vi "Opt_ROI.vi"(8 "error in (no error)":errorcluster, 10 "Number of Pre-Process Frames":i32, 11 "LTRBC":dbl[][](array[numeric])) -> (0 "error out":errorcluster, 2 "Y Centroid":dbl, 3 "ROI Out":T1 {"Contours"."Type" items=["No Selection", "Point", "Line", "Rectangle", "Oval", "Polygon", "Freehand Region", "Annulus", "Unused2", "Unused3", "Broken Line", "Freehand Line", "Rotated Rectangle"]})   [LabVIEW 2014]
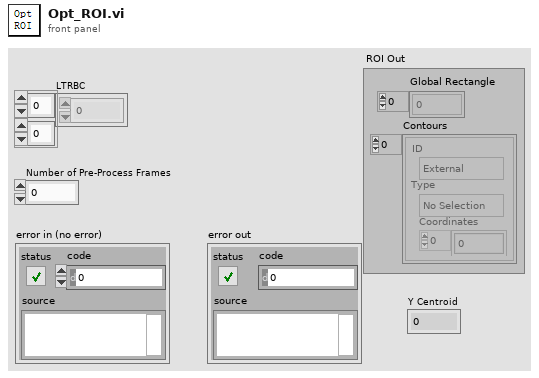
[diagram p1: front panel]
types:
  T1 = typedef "ROI Descriptor" = cluster{"Global Rectangle":i32[], "Contours":cluster{"ID":enum32{"External", "Internal"}, "Type":u32, "Coordinates":i32[]}[]}
  T2 = typedef "IMAQ Rectangle" = cluster{"Left":i32, "Top":i32, "Right":i32, "Bottom":i32, "Rotation":dbl}
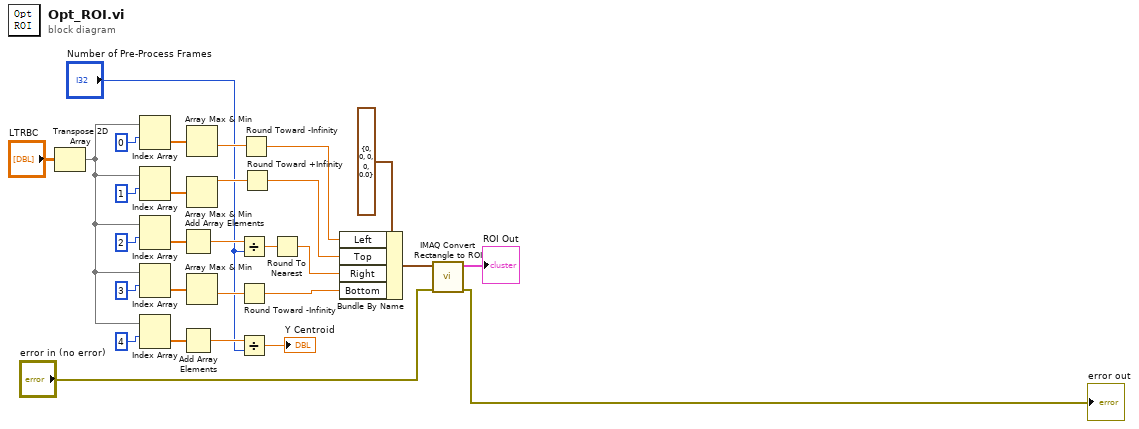
[diagram p0: block diagram]
diagram:
  n1 = Transpose 2D Array(2D array="LTRBC") -> (transposed array=w3:dbl[][])
  n2 = Index Array(array=w3, index (row)=0) -> (element=w13:dbl[])  [unwired: 1 in]
  n3 = Index Array(array=w3, index (row)=1) -> (element=w14:dbl[])  [unwired: 1 in]
  n4 = Index Array(array=w3, index (row)=2) -> (element=w15:dbl[])  [unwired: 1 in]
  n5 = Index Array(array=w3, index (row)=3) -> (element=w16:dbl[])  [unwired: 1 in]
  n6 = Index Array(array=w3, index (row)=4) -> (element=w5:dbl[])  [unwired: 1 in]
  n7 = Add Array Elements(numeric array=w15) -> (sum=w17:dbl)
  n8 = Add Array Elements(numeric array=w5) -> (sum=w6:dbl)
  n9 = Array Max & Min(array=w13) -> (min value=w19:dbl)  [unwired: 3 out]
  n10 = Array Max & Min(array=w14) -> (max value=w21:dbl)  [unwired: 3 out]
  n11 = Array Max & Min(array=w16) -> (min value=w20:dbl)  [unwired: 3 out]
  n12 = Divide(x=w17, y="Number of Pre-Process Frames") -> (x/y=w18:dbl)
  n13 = Round Toward -Infinity(1:w20) -> (0:w27:dbl)
  n14 = Divide(x=w6, y="Number of Pre-Process Frames") -> (x/y=→"Y Centroid":dbl)
  n15 = Round Toward -Infinity(1:w19) -> (0:w24:dbl)
  n16 = Round Toward +Infinity(x=w21) -> (ceil(x): smallest int >= x=w25:dbl)
  n17 = Round To Nearest(number=w18) -> (nearest integer value=w26:dbl)
  n18 = Bundle By Name(cluster=T2 {"Left"=0, "Top"=0, "Right"=0, "Bottom"=0, "Rotation"=0.0} ("Rectangle"), "Left"=w24, "Top"=w25, "Right"=w26, "Bottom"=w27) -> (w23:T2)
  n19 = call "IMAQ Convert Rectangle to ROI"("error in (no error)"="error in (no error)", "Rectangle"=w23) -> ("error out"=→"error out":errorcluster, "ROI Descriptor"=→"ROI Out":T1)  [unwired: 7 in]
